vi "DMS_main_VI_BM.vi"(0 "Elution Progress Bar Refnum":refnum<vi>, 1 "Elution Countdown Timer Refnum":refnum<vi>, 2 "Sparging Progress Bar Refnum":refnum<vi>, 3 "Sparging Countdown Timer Refnum":refnum<vi>, 4 "Temp Refnum":refnum<vi>, 5 "Skip sample handling":bool, 6 "Current Analyte Refnum":refnum<vi>, 7 "Metadata":T1={"Local save location:"="C:\\Users\\bcamc\\OneDrive\\Desktop\\LabVIEW\\Test_metadata", "Cruise ID"="LaPerouse", "Sampling Timestamp"="2023-07-19 15:23:13", "Elution Timestamp"="2023-07-19 15:29:12", "GPS_Latitude"=-999.0, "GPS_Longitude"=-999.0, "DMS_std_conc"=0.0, "DMSP_std_conc"=0.0, "DMSO_std_conc"=0.0, "Std_index"=0.0, "Initial Trap Temp (oC)"=174.0, "Max Trap Temp (oC)"=174.0, "Final Trap Temp (oC)"=0.0, "Flow Rate (mL/min)"=0.0, "Comment"="", "GPS_Minute"=-999.0, "GPS_Day"=-999.0, "GPS_jd"=-999.0, "GPS_Hour"=-999.0, "GPS_Second"=-999.0, "GPS Baud"=4800.0, "COM Port (GPS)"="COM10", "Use GPS?"=FALSE, "Format Date"="%d-%d-%d"} {"GPS_Latitude" format="%_4g"; "GPS_Longitude" format="%_4g"; "GPS_jd" format="%_5g"; "Std_index" format="%.2g"; "DMSO_std_conc" format="%.2f"; "DMSP_std_conc" format="%.2f"; "DMS_std_conc" format="%.2f"}, 8 "Analysis Type":T3(ring), 9 "Pump Parameters":T4={"Speed 1"="100", "Speed 2"="250", "Speed 3"="450", "Speed 4"="250", "UW/Sample"="5", "Sparge"="2", "Std"="4", "Waste"="15", "Air"="14", "Milli-Q"="1", "H2SO4"="6", "NaOH"="3", "Catalyst"="7", "Cell (H+ side)"="8", "Cell (sample side)"="9", "NaCl"="11"}, 10 "Sample Params":T6={"DMS Sparge Time (min)"=7.0, "Elution Time (min)"=1.5, "COM port (16 Pos. Valve)"="COM10", "Trap Heating Time (ms)"=675.0, "COM Port (DC Power)"="COM11", "COM Port (Runze)"="COM12", "sample volume"=10.0, "DMSO red. Sparge Time  (min)"=32.0, "DMSO Red. Duration (min)"=30.0, "Bypass sample handling (debugging)"=FALSE, "Reverse Reduction?"=FALSE, "Voltage (V)"="4.0", "DMSP Hydrolysis Time (min)"=13.0}, 11 "Constants":T5={"step to ml"=1920.0, "BoardNum"=1, "PosA BitNum"=6, "PosB BitNum"=5, "Heat Pulse Delay (ms)"=0.0, "Heating Iterations"=8, "N rinses"=2, "Dissolution Time (s)"=120, "SpargeBit"=0, "Extra Milli-Q (ml)"=2.0, "Valco Port Number"=6, "BitNum (Thermocouple)"=0, "Total Vol. (mL)"=12.0, "N syringe rinses"=2, "NaOH Vol (ml)"=2.0, "FanBit"=0}) -> ()   [LabVIEW 2021]
uses:
  SubVIs/Refnum_control_global_BM.vi
  SubVIs/DMS-related/Sparge_stop.vi
  SubVIs/Plot_trap_heating_global_BM.vi
  SubVIs/DMS-related/Elution_stop.vi
  SubVIs/DMSO-related/Temp_global_BM.vi
panel:
  out "Current Analysis":string
  in  "Mode Selection":T2(ring)
  out "Elution Countdown (min)":dbl=-0.0013020833333333333 format="%.2f"
  out "Elution Progress Bar":u8(slide)=100 scale=0.0..100.0
  out "Error out":errorcluster
  out "Temp (oC)":i32=174
  in  "Error in":errorcluster
  out "Heating":bool
  out "Drying Flow":bool
  out "Sparging":bool
  out "Sparge Countdown (min)":dbl=-0.00078125 format="%.2g"
  out "Sparging Progress Bar":u8(slide)=100 scale=0.0..100.0
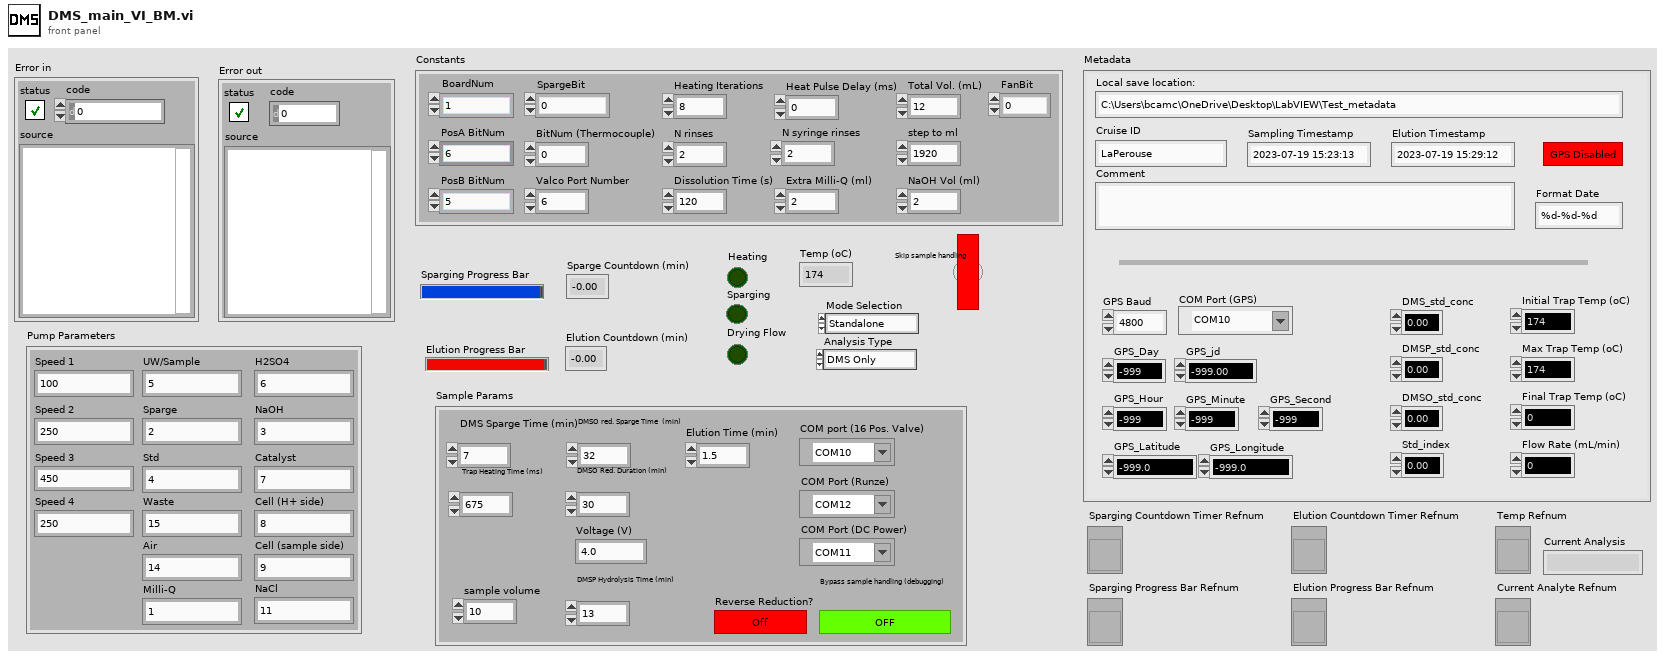
[diagram p1: front panel]
types:
  T1 = cluster{"Local save location:":string, "Cruise ID":string, "Sampling Timestamp":string, "Elution Timestamp":string, "GPS_Latitude":dbl, "GPS_Longitude":dbl, "DMS_std_conc":dbl, "DMSP_std_conc":dbl, "DMSO_std_conc":dbl, "Std_index":dbl, "Initial Trap Temp (oC)":dbl, "Max Trap Temp (oC)":dbl, "Final Trap Temp (oC)":dbl, "Flow Rate (mL/min)":dbl, "Comment":string, "GPS_Minute":dbl, "GPS_Day":dbl, "GPS_jd":dbl, "GPS_Hour":dbl, "GPS_Second":dbl, "GPS Baud":dbl, "COM Port (GPS)":refnum<visa-resource-name>, "Use GPS?":bool, "Format Date":string}
  T2 = enum16{"Standalone", "Standard Curve", "Point Std", "Analysis"}
  T3 = enum16{"DMS Only", "DMS/O", "DMS/P", "DMS/O/P", "DMSO Only"}
  T4 = cluster{"Speed 1":string, "Speed 2":string, "Speed 3":string, "Speed 4":string, "UW/Sample":string, "Sparge":string, "Std":string, "Waste":string, "Air":string, "Milli-Q":string, "H2SO4":string, "NaOH":string, "Catalyst":string, "Cell (H+ side)":string, "Cell (sample side)":string, "NaCl":string}
  T5 = cluster{"step to ml":dbl, "BoardNum":u32, "PosA BitNum":u32, "PosB BitNum":u32, "Heat Pulse Delay (ms)":dbl, "Heating Iterations":i32, "N rinses":i32, "Dissolution Time (s)":u32, "SpargeBit":u32, "Extra Milli-Q (ml)":dbl, "Valco Port Number":i32, "BitNum (Thermocouple)":u32, "Total Vol. (mL)":dbl, "N syringe rinses":i32, "NaOH Vol (ml)":dbl, "FanBit":u32}
  T6 = cluster{"DMS Sparge Time (min)":dbl, "Elution Time (min)":dbl, "COM port (16 Pos. Valve)":refnum<visa-resource-name>, "Trap Heating Time (ms)":dbl, "COM Port (DC Power)":refnum<visa-resource-name>, "COM Port (Runze)":refnum<visa-resource-name>, "sample volume":dbl, "DMSO red. Sparge Time  (min)":dbl, "DMSO Red. Duration (min)":dbl, "Bypass sample handling (debugging)":bool, "Reverse Reduction?":bool, "Voltage (V)":string, "DMSP Hydrolysis Time (min)":dbl}
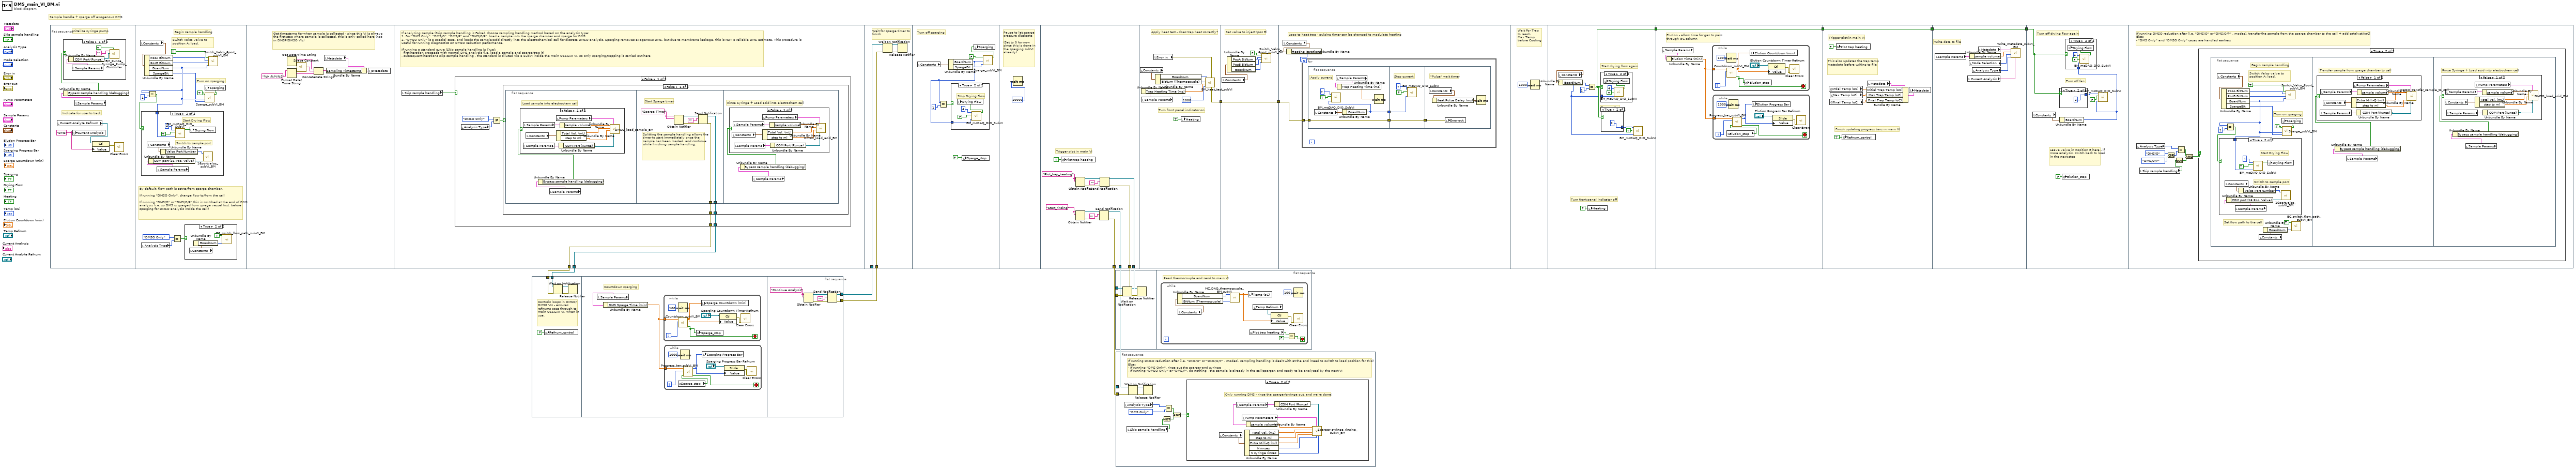
[diagram p0: block diagram]
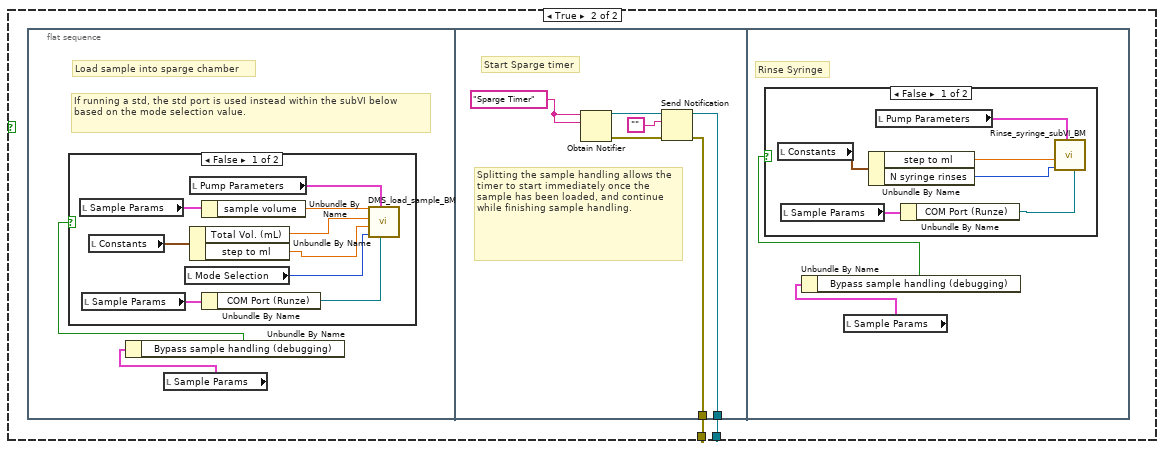
[diagram p8: hidden frame]
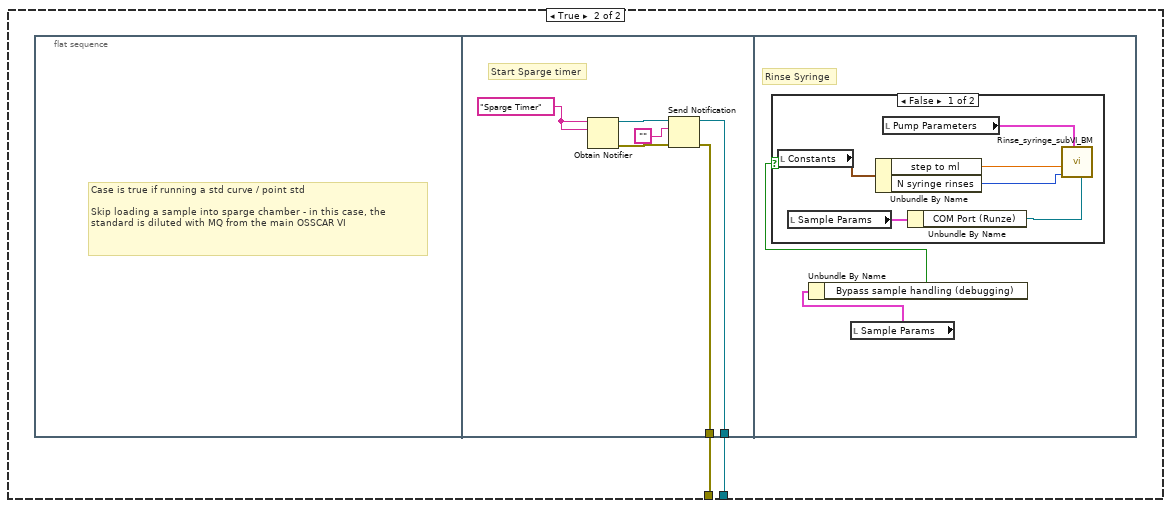
[diagram p11: hidden frame]
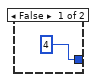
[diagram p14: hidden frame]
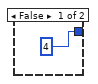
[diagram p16: hidden frame]
diagram:
  # "Sample handle + sparge off exogenous DMS"
  n1 = flat-sequence {
    tunnel: [w57] -> w9
    tunnel: [w56] -> w1
    tunnel: w10 -> [w136]
    tunnel: w11 -> [w135]
    tunnel: [w158] -> w5
    tunnel: [w157] -> w4
    tunnel: [w152] -> w3
    tunnel: [w151] -> w2
    tunnel: [w172] -> w14
    tunnel: [w177] -> w13
    tunnel: w14 -> [w177]
    tunnel: w13 -> [w181]
    tunnel: [w206] -> w12
    tunnel: w12 -> [w216]
    tunnel: [w216] -> w8
    tunnel: w8 -> [w239]
    tunnel: [w239] -> w7
    tunnel: w7 -> [w246]
    tunnel: [w246] -> w6
    tunnel: w6 -> [w251]
    frame #0 {
      w16 = "DMS" ("Current Analysis")
      # "Indicate for user to track"
      # "Initalize syringe pump"
      n2 = local read "Current Analyte Refnum"() -> (w17:refnum<vi>)
      n3 = local write "Current Analysis"(w16) -> ()
      n4 = local read "Sample Params"() -> (w18:T6)
      n5 = Unbundle By Name(w18) -> ("Bypass sample handling (debugging)"=w19:bool)
      n6 = case shown="False" w19 {
        frame False {
          n7 = local read "Sample Params"() -> (w20:T6)
          n8 = Unbundle By Name(w20) -> ("COM Port (Runze)"=w21:refnum<visa-resource-name>)
          n9 = call "BM_Runze_Syringe_Pump_Controller.vi"("Initialize Plunger?"=TRUE ("Initialize?"), "COM Port (Runze)"=w21, "Enter Command"="") -> ()  [unwired: 6 in, 3 out]
        }
        frame True {
        }
      }
      n10 = property class="Ctl"(reference=w17, "Value"=w16) -> (error out=w15:errorcluster)  [unwired: 1 in, 1 out]
      n11 = call <vilib>:"Clear Errors.vi"("error in (no error)"=w15) -> ()  [unwired: 5 in, 2 out]
    }
    frame #1 {
      # "By default, flow path is set to/from sparge chamber.\n\nIf running \"DMSO Only\", change flow to/from the cell\n\nIf running \"DMS/O\" or \"DMS/O/P\" this is switched at the end of DMS analysis (i.e. so DMS is sparged from sprage vessel first, before sparging for DMSO analysis inside the cell)"
      # "Turn on sparging."
      # "Switch Valco valve to position A: load."
      # "Begin sample handling"
      n12 = local read "Constants"() -> (w34:T5)
      n13 = local read "Analysis Type"() -> (w26:T3)
      n14 = Unbundle By Name(w34) -> ("PosA BitNum"=w33:u32, "PosB BitNum"=w32:u32, "BoardNum"=w31:u32, "SpargeBit"=w30:u32)
      n15 = Equal?(x=w31, y=u32 1) -> (x = y?=w36:bool)
      n16 = case shown="True" w36 {
        tunnel: w31 -> [_ w44]
        frame False {
        }
        frame True {
          # "Switch to sample port"
          # "Start Drying Flow"
          n17 = local read "Constants"() -> (w42:T5)
          n18 = local read "Sample Params"() -> (w40:T6)
          n19 = Unbundle By Name(w40) -> ("COM port (16 Pos. Valve)"=w41:refnum<visa-resource-name>)
          n20 = Unbundle By Name(w42) -> ("Valco Port Number"=w43:i32)
          n21 = call "BM_mcDAQ_DIO_SubVI.vi"("BoardNum"=w44, "BitValue"=TRUE, "BitNum"=4) -> ("Control out"=w47:bool)  [unwired: 8 in]
          n22 = local write "Drying Flow"(w47) -> ()
          n23 = call "16portvalco_subVI_BM.vi"("COM Port (16 Pos. Valve)"=w41, "Port Number"=w43) -> ()  [unwired: 9 in, 1 out]
        }
      }
      n24 = Equal?(x=T3."DMSO Only", y=w26) -> (x = y?=w24:bool)
      n25 = case shown="True" w24 {
        frame False {
        }
        frame True {
          n26 = local read "Constants"() -> (w38:T5)
          n27 = Unbundle By Name(w38) -> ("BoardNum"=w39:u32)
          n28 = call "EC_switch_flow_path_subVI_BM.vi"("BoardNum"=w39, "Switch Flow Path"=TRUE) -> ()  [unwired: 10 in]
        }
      }
      n29 = call "Sparge_subVI_BM.vi"("BitNum"=w30, "BoardNum"=w31, "Sparge now"=TRUE) -> ("Sparging"=w35:bool)  [unwired: 8 in]
      n30 = local write "Sparging"(w35) -> ()
      n31 = call "Switch_Valco_6port_subVI_BM.vi"("Load (T) or Inject (F)"=TRUE, "PosA BitNum"=w33, "PosB BitNum"=w32, "BoardNum"=w31) -> ()  [unwired: 6 in, 1 out]
    }
    frame #2 {
      # "Get timestamp for when sample is collected - since this VI is always the first step where sample is collected, this is only called here (not in DMSP/DMSO VIs)"
      n32 = Get Date/Time String() -> (date string=w51:string)  [unwired: 3 in, 1 out]
      n33 = Format Date/Time String(time format string (%c)="%H:%M:%S" ("format string")) -> (date/time string=w50:string)  [unwired: 2 in]
      n34 = call <vilib>:"Space Constant.vi"() -> ("String"=w49:string)
      n35 = Concatenate Strings(w51, w49, w50) -> (w53:string)
      n36 = local read "Metadata"() -> (w52:T1)
      n37 = Bundle By Name(cluster=w52, "Sampling Timestamp"=w53) -> (w54:T1)
      n38 = local write "Metadata"(w54) -> ()
    }
    frame #3 {
      # "If analyzing sample (Skip sample handling is False), choose sampling handling method based on the analysis type:\n1. For \"DMS Only\", \"DMS/O\", \"DMS/P\" and \"DMS/O/P\", load a sample into the sparge chamber and sparge for DMS\n2. \"DMSO Only\" is a special case, and loads the sample/acid directly into the electrochemical cell for discrete DMSO analysis. Sparging removes exogenous DMS, but due to membrane leakage, this is NOT a reliable DMS estimate. This procedure is useful for running diagnostics on DMSO reduction performance.\n\nIf running a standard curve (Skip sample handling is True):\n- first iteration proceeds with normal DMS analysis (i.e. load a sample and sparge/trap it)\n- subsequent iterations skip sample handling - the standard is diluted via a SubVI inside the main OSSCAR VI, so only sparging/trapping is carried out here"
      n39 = local read "Skip sample handling"() -> (w55:bool)
      n40 = case shown="False" w55 {
        tunnel: [w62 w119] -> w57
        tunnel: [w58 w118] -> w56
        frame False {
          n41 = local read "Analysis Type"() -> (w61:T3)
          n42 = Not Equal?(x=T3."DMSO Only", y=w61) -> (x != y?=w59:bool)
          n43 = case shown="False" w59 {
            tunnel: [w64 w91] -> w62
            tunnel: [w63 w92] -> w58
            frame False {
              n44 = flat-sequence {
                tunnel: [w76] -> w64
                tunnel: [w75] -> w63
                frame #0 {
                  # "Load sample into electrochem cell"
                  n45 = local read "Sample Params"() -> (w65:T6)
                  n46 = Unbundle By Name(w65) -> ("Bypass sample handling (debugging)"=w66:bool)
                  n47 = case shown="False" w66 {
                    frame False {
                      n48 = local read "Sample Params"() -> (w68:T6)
                      n49 = local read "Sample Params"() -> (w70:T6)
                      n50 = local read "Constants"() -> (w73:T5)
                      n51 = local read "Pump Parameters"() -> (w74:T4)
                      n52 = Unbundle By Name(w73) -> ("Total Vol. (mL)"=w72:dbl, "step to ml"=w71:dbl)
                      n53 = Unbundle By Name(w68) -> ("COM Port (Runze)"=w67:refnum<visa-resource-name>)
                      n54 = Unbundle By Name(w70) -> ("sample volume"=w69:dbl)
                      n55 = call "DMSO_load_sample_BM.vi"("COM Port"=w67, "Pump Parameters"=w74, "step to ml"=w71, "Total Vol. (mL)"=w72, "Sample Vol. (mL)"=w69) -> ()  [unwired: 7 in]
                    }
                    frame True {
                    }
                  }
                }
                frame #1 {
                  w77 = "Sparge Timer"
                  # "Splitting the sample handling allows the timer to start immediately once the sample has been loaded, and continue while finishing sample handling."
                  # "Start Sparge timer"
                  n56 = Obtain Notifier(name (unnamed)=w77, notification data type=w77) -> (notifier out=w79:refnum<notifier>, error out=w80:errorcluster)  [unwired: 2 in, 1 out]
                  n57 = Send Notification(notification="", notifier=w79, error in (no error)=w80) -> (notifier out=w76:refnum<notifier>, error out=w75:errorcluster)
                }
                frame #2 {
                  # "Rinse Syringe + Load acid into electrochem cell"
                  n58 = local read "Sample Params"() -> (w81:T6)
                  n59 = Unbundle By Name(w81) -> ("Bypass sample handling (debugging)"=w82:bool)
                  n60 = case shown="False" w82 {
                    frame False {
                      n61 = local read "Constants"() -> (w89:T5)
                      n62 = local read "Sample Params"() -> (w86:T6)
                      n63 = local read "Sample Params"() -> (w85:T6)
                      n64 = local read "Pump Parameters"() -> (w90:T4)
                      n65 = Unbundle By Name(w89) -> ("Total Vol. (mL)"=w88:dbl, "step to ml"=w87:dbl)
                      n66 = Unbundle By Name(w86) -> ("sample volume"=w83:dbl)
                      n67 = Unbundle By Name(w85) -> ("COM Port (Runze)"=w84:refnum<visa-resource-name>)
                      n68 = call "DMSO_load_acid_BM.vi"("COM Port"=w84, "Pump Parameters"=w90, "step to ml"=w87, "Total Vol. (mL)"=w88, "Sample Vol. (mL)"=w83) -> ()  [unwired: 7 in]
                    }
                    frame True {
                    }
                  }
                }
              }
            }
            frame True {
              n69 = flat-sequence {
                tunnel: [w105] -> w91
                tunnel: [w104] -> w92
                frame #0 {
                  # "If running a std, the std port is used instead within the subVI below based on the mode selection value."
                  # "Load sample into sparge chamber"
                  n70 = local read "Sample Params"() -> (w93:T6)
                  n71 = Unbundle By Name(w93) -> ("Bypass sample handling (debugging)"=w94:bool)
                  n72 = case shown="False" w94 {
                    frame False {
                      n73 = local read "Sample Params"() -> (w99:T6)
                      n74 = local read "Sample Params"() -> (w97:T6)
                      n75 = local read "Constants"() -> (w102:T5)
                      n76 = local read "Mode Selection"() -> (w95:T2)
                      n77 = local read "Pump Parameters"() -> (w103:T4)
                      n78 = Unbundle By Name(w102) -> ("Total Vol. (mL)"=w101:dbl, "step to ml"=w100:dbl)
                      n79 = Unbundle By Name(w99) -> ("sample volume"=w98:dbl)
                      n80 = Unbundle By Name(w97) -> ("COM Port (Runze)"=w96:refnum<visa-resource-name>)
                      n81 = call "DMS_load_sample_BM.vi"("COM Port"=w96, "Pump Parameters"=w103, "Mode Selection"=w95, "step to ml"=w100, "Total Vol. (mL)"=w101, "Sample Vol. (mL)"=w98) -> ()  [unwired: 6 in]
                    }
                    frame True {
                    }
                  }
                }
                frame #1 {
                  w106 = "Sparge Timer"
                  # "Splitting the sample handling allows the timer to start immediately once the sample has been loaded, and continue while finishing sample handling."
                  # "Start Sparge timer"
                  n82 = Obtain Notifier(name (unnamed)=w106, notification data type=w106) -> (notifier out=w108:refnum<notifier>, error out=w109:errorcluster)  [unwired: 2 in, 1 out]
                  n83 = Send Notification(notification="", notifier=w108, error in (no error)=w109) -> (notifier out=w105:refnum<notifier>, error out=w104:errorcluster)
                }
                frame #2 {
                  # "Rinse Syringe"
                  n84 = local read "Sample Params"() -> (w110:T6)
                  n85 = Unbundle By Name(w110) -> ("Bypass sample handling (debugging)"=w111:bool)
                  n86 = case shown="False" w111 {
                    frame False {
                      n87 = local read "Constants"() -> (w116:T5)
                      n88 = local read "Sample Params"() -> (w114:T6)
                      n89 = Unbundle By Name(w116) -> ("step to ml"=w115:dbl, "N syringe rinses"=w112:i32)
                      n90 = local read "Pump Parameters"() -> (w117:T4)
                      n91 = Unbundle By Name(w114) -> ("COM Port (Runze)"=w113:refnum<visa-resource-name>)
                      n92 = call "Rinse_syringe_subVI_BM.vi"("COM Port"=w113, "Pump Parameters"=w117, "N syringe rinses"=w112, "step to ml"=w115) -> ()  [unwired: 8 in]
                    }
                    frame True {
                    }
                  }
                }
              }
            }
          }
        }
        frame True {
          n93 = flat-sequence {
            tunnel: [w121] -> w119
            tunnel: [w120] -> w118
            frame #0 {
              # "Case is true if running a std curve / point std\n\nSkip loading a sample into sparge chamber - in this case, the standard is diluted with MQ from the main OSSCAR VI"
            }
            frame #1 {
              w122 = "Sparge Timer"
              # "Start Sparge timer"
              n94 = Obtain Notifier(name (unnamed)=w122, notification data type=w122) -> (notifier out=w124:refnum<notifier>, error out=w125:errorcluster)  [unwired: 2 in, 1 out]
              n95 = Send Notification(notification="", notifier=w124, error in (no error)=w125) -> (notifier out=w121:refnum<notifier>, error out=w120:errorcluster)
            }
            frame #2 {
              # "Rinse Syringe"
              n96 = local read "Sample Params"() -> (w126:T6)
              n97 = Unbundle By Name(w126) -> ("Bypass sample handling (debugging)"=w127:bool)
              n98 = case shown="False" w127 {
                frame False {
                  n99 = local read "Constants"() -> (w132:T5)
                  n100 = local read "Sample Params"() -> (w130:T6)
                  n101 = Unbundle By Name(w132) -> ("step to ml"=w131:dbl, "N syringe rinses"=w128:i32)
                  n102 = local read "Pump Parameters"() -> (w133:T4)
                  n103 = Unbundle By Name(w130) -> ("COM Port (Runze)"=w129:refnum<visa-resource-name>)
                  n104 = call "Rinse_syringe_subVI_BM.vi"("COM Port"=w129, "Pump Parameters"=w133, "N syringe rinses"=w128, "step to ml"=w131) -> ()  [unwired: 8 in]
                }
                frame True {
                }
              }
            }
          }
        }
      }
    }
    frame #4 {
      # "Wait for sparge timer to finish"
      n105 = Wait on Notification(notifier=w136, error in (no error)=w135) -> (notifier out=w134:refnum<notifier>, error out=w137:errorcluster)  [unwired: 4 out]
      n106 = Release Notifier(notifier=w134, error in (no error)=w137) -> ()  [unwired: 1 in, 3 out]
    }
    frame #5 {
      # "Turn off sparging"
      n107 = local read "Constants"() -> (w140:T5)
      n108 = Unbundle By Name(w140) -> ("BoardNum"=w138:u32, "SpargeBit"=w139:u32)
      n109 = Equal?(x=w138, y=u32 1) -> (x = y?=w143:bool)
      n110 = case shown="True" w143 {
        tunnel: w138 -> [_ w146]
        frame False {
        }
        frame True {
          # "Stop Drying Flow"
          n111 = call "BM_mcDAQ_DIO_SubVI.vi"("BoardNum"=w146, "BitValue"=FALSE, "BitNum"=4) -> ("Control out"=w147:bool)  [unwired: 8 in]
          n112 = local write "Drying Flow"(w147) -> ()
        }
      }
      n113 = global write "Sparge_stop.vi" "Sparge_stop"(FALSE ("Stop_Reached")) -> ()
      n114 = call "Sparge_subVI_BM.vi"("BitNum"=w139, "BoardNum"=w138, "Sparge now"=FALSE) -> ("Sparging"=w142:bool)  [unwired: 8 in]
      n115 = local write "Sparging"(w142) -> ()
    }
    frame #6 {
      # "Pause to let sparge\npressure dissipate\n\n(Set to 0 for now since this is done in the sparging subVI already)"
      n116 = Wait (ms)(milliseconds to wait=10000) -> ()  [unwired: 1 out]
    }
    frame #7 {
      w153 = "Start_rinsing"
      w160 = "Plot_trap_heating"
      # "Trigger plot in main VI"
      n117 = global write "Plot_trap_heating_global_BM.vi" "Plot trap heating"(TRUE ("Plot trap heating")) -> ()
      n118 = Obtain Notifier(name (unnamed)=w153, notification data type=w153) -> (notifier out=w156:refnum<notifier>, error out=w155:errorcluster)  [unwired: 2 in, 1 out]
      n119 = Obtain Notifier(name (unnamed)=w160, notification data type=w160) -> (notifier out=w163:refnum<notifier>, error out=w162:errorcluster)  [unwired: 2 in, 1 out]
      n120 = Send Notification(notification="", notifier=w156, error in (no error)=w155) -> (notifier out=w152:refnum<notifier>, error out=w151:errorcluster)
      n121 = Send Notification(notification="", notifier=w163, error in (no error)=w162) -> (notifier out=w158:refnum<notifier>, error out=w157:errorcluster)
    }
    frame #8 {
      # "Turn front panel indicator on"
      # "Apply heat test - does trap heat correctly?"
      n122 = local read "Constants"() -> (w168:T5)
      n123 = local read "Sample Params"() -> (w166:T6)
      n124 = Unbundle By Name(w166) -> ("Trap Heating Time (ms)"=w165:dbl)
      n125 = local read "Error in"() -> (w171:errorcluster)
      n126 = Unbundle By Name(w168) -> ("BoardNum"=w167:u32, "BitNum (Thermocouple)"=w164:u32)
      n127 = local write "Heating"(TRUE ("Heating")) -> ()
      n128 = call "BM_heat_test_subVI.vi"("error in (no error)"=w171, "Heat Pulse Delay (ms)"=u32 1000, "Trap Heating Time (ms)"=w165, "BitNum"=w164, "BoardNum"=w167) -> ("error out"=w172:errorcluster)  [unwired: 6 out]
    }
    frame #9 {
      # "Set valve to inject (pos B)"
      n129 = local read "Constants"() -> (w176:T5)
      n130 = Unbundle By Name(w176) -> ("PosA BitNum"=w175:u32, "PosB BitNum"=w174:u32, "BoardNum"=w173:u32)
      n131 = call "Switch_Valco_6port_subVI_BM.vi"("Load (T) or Inject (F)"=FALSE, "PosA BitNum"=w175, "PosB BitNum"=w174, "BoardNum"=w173) -> ()  [unwired: 6 in, 1 out]
    }
    frame #10 {
      # "Loop to heat trap - pulsing timer can be changed to modulate heating"
      n132 = local read "Constants"() -> (w180:T5)
      n133 = Unbundle By Name(w180) -> ("Heating Iterations"=w179:i32)
      n134 = for {
        N: w179 -> [_]
        tunnel: w181 -> [w185]
        n135 = flat-sequence {
          tunnel: [w190] -> w183
          tunnel: [w188] -> w182
          tunnel: w185 -> [w190]
          tunnel: [w194] -> w184
          tunnel: w183 -> [w194]
          tunnel: w182 -> [w193]
          tunnel: w184 -> [w197]
          frame #0 {
            # "Apply current"
            n136 = local read "Constants"() -> (w189:T5)
            n137 = local read "Sample Params"() -> (w186:T6)
            n138 = Unbundle By Name(w186) -> ("Trap Heating Time (ms)"=w187:dbl)
            n139 = Unbundle By Name(w189) -> ("BoardNum"=w188:u32)
            n140 = call "BM_mcDAQ_DIO_SubVI.vi"("BoardNum"=w188, "BitValue"=TRUE, "BitNum"=7) -> ()  [unwired: 8 in, 1 out]
            n141 = Wait (ms)(milliseconds to wait=w187) -> ()  [unwired: 1 out]
          }
          frame #1 {
            # "Stop current"
            n142 = call "BM_mcDAQ_DIO_SubVI.vi"("BoardNum"=w193, "BitValue"=FALSE, "BitNum"=7) -> ()  [unwired: 8 in, 1 out]
          }
          frame #2 {
            # "\"Pulse\" wait timer"
            n143 = local read "Constants"() -> (w199:T5)
            n144 = Unbundle By Name(w199) -> ("Heat Pulse Delay (ms)"=w198:dbl)
            n145 = local write "Error out"(w197) -> ()
            n146 = Wait (ms)(milliseconds to wait=w198) -> ()  [unwired: 1 out]
          }
        }
      }
    }
    frame #11 {
      # "Wait For Trap\nto reach\nMax Temp \nbefore Cooling"
      n147 = Wait (ms)(milliseconds to wait=1000) -> ()  [unwired: 1 out]
    }
    frame #12 {
      # "Turn on fan"
      # "Turn front panel indicator off"
      # "Start drying flow again"
      n148 = local read "Constants"() -> (w202:T5)
      n149 = Unbundle By Name(w202) -> ("BoardNum"=w201:u32)
      n150 = Equal?(x=w201, y=u32 1) -> (x = y?=w206:bool)
      n151 = local write "Heating"(FALSE ("Heating")) -> ()
      n152 = case shown="True" w206 {
        tunnel: w201 -> [_ w211]
        frame False {
        }
        frame True {
          n153 = call "BM_mcDAQ_DIO_SubVI.vi"("BoardNum"=w211, "BitValue"=TRUE, "BitNum"=u32 4) -> ("Control out"=w210:bool)  [unwired: 8 in]
          n154 = local write "Drying Flow"(w210) -> ()
        }
      }
      n155 = case shown="True" w206 {
        tunnel: [u32 4 ("BitNum") u32 2 ("BitNum")] -> w204
        frame False {
        }
        frame True {
        }
      }
      n156 = call "BM_mcDAQ_DIO_SubVI.vi"("BoardNum"=w201, "BitValue"=TRUE, "BitNum"=w204) -> ()  [unwired: 8 in, 1 out]
    }
    frame #13 {
      # "Elution - allow time for gas to pass through GC column"
      n157 = local read "Sample Params"() -> (w215:T6)
      n158 = Unbundle By Name(w215) -> ("Elution Time (min)"=w214:dbl)
      n159 = while {
        tunnel: w214 -> [w226]
        i -> [w230]
        stop <- w229 stop-if-true
        n160 = Wait (ms)(milliseconds to wait=u32 100) -> ()  [unwired: 1 out]
        n161 = call "Countdown_subVI_BM.vi"("Current Iteration"=w230, "Runtime (min)"=w226) -> ("Global Stop"=w229:bool, "Countdown Timer (min)"=w227:dbl)  [unwired: 8 in]
        n162 = global write "Elution_stop.vi" "Elution_stop"(w229) -> ()
        n163 = local write "Elution Countdown (min)"(w227) -> ()
        n164 = property class="Ctl"(reference="Elution Countdown Timer Refnum", "Value"=w227) -> (error out=w225:errorcluster)  [unwired: 1 in, 1 out]
        n165 = call <vilib>:"Clear Errors.vi"("error in (no error)"=w225) -> ()  [unwired: 5 in, 2 out]
      }
      n166 = while {
        tunnel: w214 -> [w218]
        i -> [w223]
        stop <- w221 stop-if-true
        n167 = global read "Elution_stop.vi" "Elution_stop"() -> (w222:bool)
        n168 = Wait (ms)(milliseconds to wait=u32 1000) -> ()  [unwired: 1 out]
        n169 = call "Progress_bar_subVI_BM.vi"("Global Stop"=w222, "Current Iteration"=w223, "Runtime (min)"=w218) -> ("Loop Stop"=w221:bool, "Progress Bar"=w219:u8)  [unwired: 7 in]
        n170 = local write "Elution Progress Bar"(w219) -> ()
        n171 = property class="Slide"(reference="Elution Progress Bar Refnum", "Value"=w219) -> (error out=w217:errorcluster)  [unwired: 1 in, 1 out]
        n172 = call <vilib>:"Clear Errors.vi"("error in (no error)"=w217) -> ()  [unwired: 5 in, 2 out]
      }
    }
    frame #14 {
      # "Finish updating progress bars in main VI"
      # "This also updates the trap temp metadata before writing to file"
      # "Trigger plot in main VI"
      n173 = global read "Temp_global_BM.vi" "Intial Temp (oC)"() -> (w235:dbl)
      n174 = global read "Temp_global_BM.vi" "Final Temp (oC)"() -> (w237:dbl)
      n175 = global read "Temp_global_BM.vi" "Max Temp (oC)"() -> (w236:dbl)
      n176 = global write "Plot_trap_heating_global_BM.vi" "Plot trap heating"(FALSE ("Plot trap heating")) -> ()
      n177 = global write "Refnum_control_global_BM.vi" "Refnum_control"(TRUE ("Refnum_control")) -> ()
      n178 = local read "Metadata"() -> (w233:T1)
      n179 = Bundle By Name(cluster=w233, "Initial Trap Temp (oC)"=w235, "Max Trap Temp (oC)"=w236, "Final Trap Temp (oC)"=w237) -> (w234:T1)
      n180 = local write "Metadata"(w234) -> ()
    }
    frame #15 {
      # "Write data to file"
      n181 = local read "Sample Params"() -> (w240:T6)
      n182 = local read "Current Analysis"() -> (w245:string)
      n183 = local read "Mode Selection"() -> (w243:T2)
      n184 = Unbundle By Name(w240) -> ("sample volume"=w242:dbl)
      n185 = local read "Analysis Type"() -> (w244:T3)
      n186 = local read "Metadata"() -> (w241:T1)
      n187 = call "Write_metadata_subVI_BM.vi"("Analyte"=w245, "Analysis Type"=w244, "Mode Selection"=w243, "sample volume"=w242, "Metadata"=w241) -> ()  [unwired: 7 in]
    }
    frame #16 {
      # "Leave valve in Position B here - if more analysis, switch back to load in the next step"
      # "Turn off fan"
      # "Turn off drying flow again"
      n188 = local read "Constants"() -> (w248:T5)
      n189 = case shown="True" w251 {
        tunnel: [u32 4 ("BitNum") u32 2 ("BitNum")] -> w250
        frame False {
        }
        frame True {
        }
      }
      n190 = Unbundle By Name(w248) -> ("BoardNum"=w247:u32)
      n191 = global write "Elution_stop.vi" "Elution_stop"(FALSE ("Elution_stop")) -> ()
      n192 = case shown="True" w251 {
        tunnel: w247 -> [_ w256]
        frame False {
        }
        frame True {
          n193 = call "BM_mcDAQ_DIO_SubVI.vi"("BoardNum"=w256, "BitValue"=FALSE, "BitNum"=u32 4) -> ("Control out"=w255:bool)  [unwired: 8 in]
          n194 = local write "Drying Flow"(w255) -> ()
        }
      }
      n195 = call "BM_mcDAQ_DIO_SubVI.vi"("BoardNum"=w247, "BitValue"=FALSE, "BitNum"=w250) -> ()  [unwired: 8 in, 1 out]
    }
    frame #17 {
      # "If running DMSO reduction after (i.e. \"DMS/O\" or \"DMS/O/P\" , modes), transfer the sample from the sparge chamber to the cell + add catalyst/NaCl\nElse:\n- \"DMS Only\" and \"DMSO Only\" cases are handled earliers"
      n196 = local read "Analysis Type"() -> (w261:T3)
      n197 = local read "Skip sample handling"() -> (w263:bool)
      n198 = Or(x=T3."DMS/O", y=T3."DMS/O/P") -> (x .or. y?=w262:i32)
      n199 = Not(x=w263) -> (.not. x?=w264:bool)
      n200 = Equal?(x=w261, y=w262) -> (x = y?=w265:bool)
      n201 = And(x=w265, y=w264) -> (x .and. y?=w266:bool)
      n202 = case shown="True" w266 {
        frame False {
        }
        frame True {
          n203 = flat-sequence {
            frame #0 {
              # "Set flow path to the cell"
              # "Turn on sparging."
              # "Switch Valco valve to position A: load."
              # "Begin sample handling"
              n204 = local read "Constants"() -> (w275:T5)
              n205 = Unbundle By Name(w275) -> ("PosA BitNum"=w276:u32, "PosB BitNum"=w277:u32, "BoardNum"=w278:u32, "SpargeBit"=w279:u32)
              n206 = Equal?(x=w278, y=u32 1) -> (x = y?=w270:bool)
              n207 = case shown="True" w270 {
                tunnel: w278 -> [_ w284]
                frame False {
                }
                frame True {
                  # "Switch to sample port"
                  # "Start Drying Flow"
                  n208 = local read "Constants"() -> (w282:T5)
                  n209 = local read "Sample Params"() -> (w280:T6)
                  n210 = Unbundle By Name(w280) -> ("COM port (16 Pos. Valve)"=w281:refnum<visa-resource-name>)
                  n211 = Unbundle By Name(w282) -> ("Valco Port Number"=w283:i32)
                  n212 = call "BM_mcDAQ_DIO_SubVI.vi"("BoardNum"=w284, "BitValue"=TRUE, "BitNum"=4) -> ("Control out"=w287:bool)  [unwired: 8 in]
                  n213 = local write "Drying Flow"(w287) -> ()
                  n214 = call "16portvalco_subVI_BM.vi"("COM Port (16 Pos. Valve)"=w281, "Port Number"=w283) -> ()  [unwired: 9 in, 1 out]
                }
              }
              n215 = local read "Constants"() -> (w268:T5)
              n216 = Unbundle By Name(w268) -> ("BoardNum"=w269:u32)
              n217 = call "Sparge_subVI_BM.vi"("BitNum"=w279, "BoardNum"=w278, "Sparge now"=TRUE) -> ("Sparging"=w274:bool)  [unwired: 8 in]
              n218 = local write "Sparging"(w274) -> ()
              n219 = call "Switch_Valco_6port_subVI_BM.vi"("Load (T) or Inject (F)"=TRUE, "PosA BitNum"=w276, "PosB BitNum"=w277, "BoardNum"=w278) -> ()  [unwired: 6 in, 1 out]
              n220 = call "EC_switch_flow_path_subVI_BM.vi"("BoardNum"=w269, "Switch Flow Path"=TRUE) -> ()  [unwired: 10 in]
            }
            frame #1 {
              # "Transfer sample from sparge chamber to cell"
              n221 = local read "Sample Params"() -> (w288:T6)
              n222 = Unbundle By Name(w288) -> ("Bypass sample handling (debugging)"=w289:bool)
              n223 = case shown="False" w289 {
                frame False {
                  n224 = local read "Sample Params"() -> (w291:T6)
                  n225 = local read "Sample Params"() -> (w293:T6)
                  n226 = local read "Constants"() -> (w296:T5)
                  n227 = Unbundle By Name(w296) -> ("Extra Milli-Q (ml)"=w295:dbl, "step to ml"=w294:dbl)
                  n228 = local read "Pump Parameters"() -> (w297:T4)
                  n229 = Unbundle By Name(w291) -> ("COM Port (Runze)"=w290:refnum<visa-resource-name>)
                  n230 = Unbundle By Name(w293) -> ("sample volume"=w292:dbl)
                  n231 = call "DMSO_transfer_sample_to_cell.vi"("COM Port"=w290, "Pump Parameters"=w297, "step to ml"=w294, "Sample Vol. (mL)"=w292, "Extra Milli-Q (ml)"=w295) -> ()  [unwired: 7 in]
                }
                frame True {
                }
              }
            }
            frame #2 {
              # "Rinse Syringe + Load acid into electrochem cell"
              n232 = local read "Sample Params"() -> (w298:T6)
              n233 = Unbundle By Name(w298) -> ("Bypass sample handling (debugging)"=w299:bool)
              n234 = case shown="False" w299 {
                frame False {
                  n235 = local read "Constants"() -> (w306:T5)
                  n236 = local read "Sample Params"() -> (w303:T6)
                  n237 = local read "Sample Params"() -> (w302:T6)
                  n238 = local read "Pump Parameters"() -> (w307:T4)
                  n239 = Unbundle By Name(w306) -> ("Total Vol. (mL)"=w305:dbl, "step to ml"=w304:dbl)
                  n240 = Unbundle By Name(w303) -> ("sample volume"=w300:dbl)
                  n241 = Unbundle By Name(w302) -> ("COM Port (Runze)"=w301:refnum<visa-resource-name>)
                  n242 = call "DMSO_load_acid_BM.vi"("COM Port"=w301, "Pump Parameters"=w307, "step to ml"=w304, "Total Vol. (mL)"=w305, "Sample Vol. (mL)"=w300) -> ()  [unwired: 7 in]
                }
                frame True {
                }
              }
            }
          }
        }
      }
    }
  }
  n243 = flat-sequence {
    tunnel: w9 -> [w310]
    tunnel: w1 -> [w309]
    tunnel: [w331] -> w10
    tunnel: [w330] -> w11
    frame #0 {
      # "Controls loops in DMSO/DMSP VIs - ensures refnums pass through to main OSSCAR VI, when in use."
      n244 = global write "Refnum_control_global_BM.vi" "Refnum_control"(FALSE ("Refnum_control")) -> ()
      n245 = Wait on Notification(notifier=w310, error in (no error)=w309) -> (notifier out=w312:refnum<notifier>, error out=w311:errorcluster)  [unwired: 4 out]
      n246 = Release Notifier(notifier=w312, error in (no error)=w311) -> ()  [unwired: 1 in, 3 out]
    }
    frame #1 {
      # "Countdown sparging"
      n247 = local read "Sample Params"() -> (w314:T6)
      n248 = Unbundle By Name(w314) -> ("DMS Sparge Time (min)"=w313:dbl)
      n249 = while {
        tunnel: w313 -> [w324]
        i -> [w328]
        stop <- w327 stop-if-true
        n250 = Wait (ms)(milliseconds to wait=u32 100) -> ()  [unwired: 1 out]
        n251 = call "Countdown_subVI_BM.vi"("Current Iteration"=w328, "Runtime (min)"=w324) -> ("Global Stop"=w327:bool, "Countdown Timer (min)"=w325:dbl)  [unwired: 8 in]
        n252 = global write "Sparge_stop.vi" "Sparge_stop"(w327) -> ()
        n253 = local write "Sparge Countdown (min)"(w325) -> ()
        n254 = property class="Ctl"(reference="Sparging Countdown Timer Refnum", "Value"=w325) -> (error out=w323:errorcluster)  [unwired: 1 in, 1 out]
        n255 = call <vilib>:"Clear Errors.vi"("error in (no error)"=w323) -> ()  [unwired: 5 in, 2 out]
      }
      n256 = while {
        tunnel: w313 -> [w316]
        i -> [w321]
        stop <- w319 stop-if-true
        n257 = global read "Sparge_stop.vi" "Sparge_stop"() -> (w320:bool)
        n258 = Wait (ms)(milliseconds to wait=u32 1000) -> ()  [unwired: 1 out]
        n259 = call "Progress_bar_subVI_BM.vi"("Global Stop"=w320, "Current Iteration"=w321, "Runtime (min)"=w316) -> ("Loop Stop"=w319:bool, "Progress Bar"=w317:u8)  [unwired: 7 in]
        n260 = local write "Sparging Progress Bar"(w317) -> ()
        n261 = property class="Slide"(reference="Sparging Progress Bar Refnum", "Value"=w317) -> (error out=w315:errorcluster)  [unwired: 1 in, 1 out]
        n262 = call <vilib>:"Clear Errors.vi"("error in (no error)"=w315) -> ()  [unwired: 5 in, 2 out]
      }
    }
    frame #2 {
      w334 = "Continue Analysis"
      n263 = Obtain Notifier(name (unnamed)=w334, notification data type=w334) -> (notifier out=w332:refnum<notifier>, error out=w333:errorcluster)  [unwired: 2 in, 1 out]
      n264 = Send Notification(notification="", notifier=w332, error in (no error)=w333) -> (notifier out=w331:refnum<notifier>, error out=w330:errorcluster)
    }
  }
  n265 = flat-sequence {
    tunnel: w5 -> [w337]
    tunnel: w4 -> [w336]
    frame #0 {
      n266 = Wait on Notification(notifier=w337, error in (no error)=w336) -> (notifier out=w339:refnum<notifier>, error out=w338:errorcluster)  [unwired: 4 out]
      n267 = Release Notifier(notifier=w339, error in (no error)=w338) -> ()  [unwired: 1 in, 3 out]
    }
    frame #1 {
      # "Read thermocouple and send to main VI"
      n268 = while {
        stop <- w342 stop-if-true
        n269 = local read "Constants"() -> (w347:T5)
        n270 = Unbundle By Name(w347) -> ("BoardNum"=w348:u32, "BitNum (Thermocouple)"=w349:u32)
        n271 = call "MC_DAQ_thermocouple_BM_subVI.vi"("BitNum"=w349, "BoardNum"=w348) -> ("Temp (oC)"=w346:dbl)  [unwired: 8 in, 1 out]
        n272 = local write "Temp (oC)"(w346) -> ()
        n273 = global read "Plot_trap_heating_global_BM.vi" "Plot trap heating"() -> (w343:bool)
        n274 = local read "Temp Refnum"() -> (w345:refnum<vi>)
        n275 = property class="Ctl"(reference=w345, "Value"=w346) -> (error out=w344:errorcluster)  [unwired: 1 in, 1 out]
        n276 = Equal?(x=w343, y=FALSE) -> (x = y?=w342:bool)
        n277 = Wait (ms)(milliseconds to wait=u32 100) -> ()  [unwired: 1 out]
        n278 = call <vilib>:"Clear Errors.vi"("error in (no error)"=w344) -> ()  [unwired: 5 in, 2 out]
      }
    }
  }
  n279 = flat-sequence {
    tunnel: w3 -> [w352]
    tunnel: w2 -> [w351]
    frame #0 {
      # "If running DMSO reduction after (i.e. \"DMS/O\" or \"DMS/O/P\" , modes), sampling handling is dealt with at the end (need to switch to load position for this)\nElse:\n- If running \"DMS Only\", rinse out the sparger and syringe\n- If running \"DMSO Only\" or \"DMS/P\", do nothing - the sample is already in the cell/sparger, and ready to be analysed by the next VI"
      n280 = local read "Analysis Type"() -> (w355:T3)
      n281 = local read "Skip sample handling"() -> (w356:bool)
      n282 = Wait on Notification(notifier=w352, error in (no error)=w351) -> (notifier out=w354:refnum<notifier>, error out=w353:errorcluster)  [unwired: 4 out]
      n283 = Release Notifier(notifier=w354, error in (no error)=w353) -> ()  [unwired: 1 in, 3 out]
      n284 = Not(x=w356) -> (.not. x?=w357:bool)
      n285 = Equal?(x=w355, y=T3."DMS Only" ("x")) -> (x = y?=w358:bool)
      n286 = And(x=w358, y=w357) -> (x .and. y?=w359:bool)
      n287 = case shown="True" w359 {
        frame False {
          # "Either running\"DMSO only\" or \"DMS/P\" modes - analysis continues in either DMSP_main or DMSO_main VIs\n\nOr\n\nIn the middle of std curve, in which case sample dilution is handled in the OSSCAR VI!"
        }
        frame True {
          # "Only running DMS - rinse the sparger/syringe out, and we're done!"
          n288 = local read "Constants"() -> (w360:T5)
          n289 = local read "Sample Params"() -> (w361:T6)
          n290 = local read "Pump Parameters"() -> (w363:T4)
          n291 = Unbundle By Name(w360) -> ("Total Vol. (mL)"=w365:dbl, "step to ml"=w366:dbl, "Extra Milli-Q (ml)"=w367:dbl, "N rinses"=w368:i32, "N syringe rinses"=w369:i32)
          n292 = Unbundle By Name(w361) -> ("sample volume"=w364:dbl)
          n293 = Unbundle By Name(w361) -> ("COM Port (Runze)"=w362:refnum<visa-resource-name>)
          n294 = call "Sparger_syringe_rinsing_subVI_BM.vi"("N syringe rinses"=w369, "COM Port"=w362, "N sparge rinses"=w368, "Pump Parameters"=w363, "Extra Milli-Q (ml)"=w367, "step to ml"=w366, "Total Vol. (mL)"=w365, "Sample Volume"=w364) -> ()  [unwired: 4 in]
        }
      }
    }
  }
